vi "IMAQ Convert ROI to Oval.vi"(7 "error in (no error)":errorcluster, 10 "ROI Descriptor":T1 {"Contours"."Type" items=["No Selection", "Point", "Line", "Rectangle", "Oval", "Polygon", "Freehand Region", "Annulus", "Unused2", "Unused3", "Broken Line", "Freehand Line", "Rotated Rectangle"]}) -> (0 "error out":errorcluster, 3 "Annulus":T2 {"End Angle" min=-90.0 max=90.0 step=1.0 format="%.2f"; "Start Angle" min=-90.0 max=90.0 step=1.0 format="%.2f"; "Center X" scale=0.0..1024.0})   [LabVIEW 2013]
doc: "Converts an ROI Descriptor to an annulus."
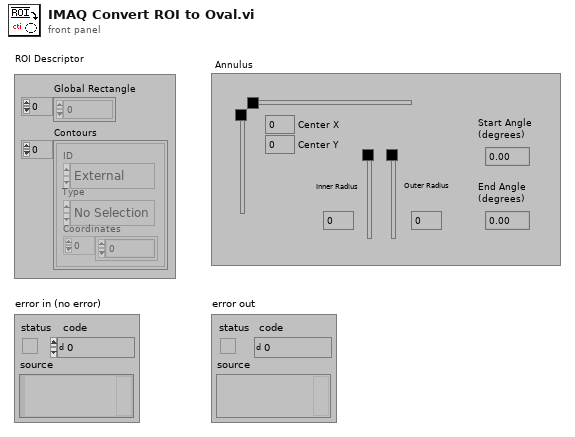
[diagram p1: front panel]
types:
  T1 = typedef "ROI Descriptor" = cluster{"Global Rectangle":i32[], "Contours":cluster{"ID":enum32{"External", "Internal"}, "Type":u32, "Coordinates":i32[]}[]}
  T2 = typedef "IMAQ Circle" = cluster{"Center X":i32, "Center Y":i32, "Inner Radius":i32, "Outer Radius":i32, "Start Angle":dbl, "End Angle":dbl}
  T3 = cluster{"ID":enum32{"External", "Internal"}, "Type":u32, "Coordinates":i32[]}[]
  T4 = cluster{"ID":enum32{"External", "Internal"}, "Type":u32, "Coordinates":i32[]}
  T5 = cluster{"Coordinates[0]":i32, "Coordinates[1]":i32, "Coordinates[2]":i32, "Coordinates[3]":i32, "Coordinates[4]":i32, "Coordinates[5]":i32}
  T6 = cluster{"Coordinates[0]":i32, "Coordinates[1]":i32, "Coordinates[2]":i32, "Coordinates[3]":i32, dbl, dbl}
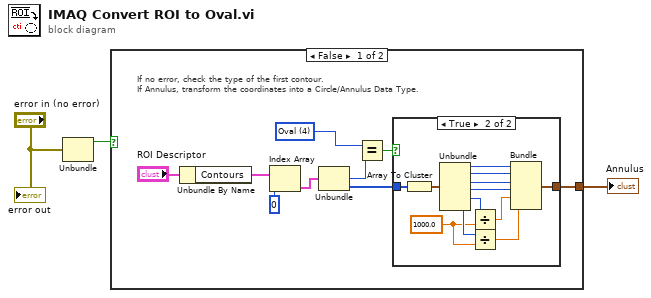
[diagram p0: block diagram]
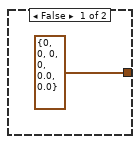
[diagram p2: hidden frame]
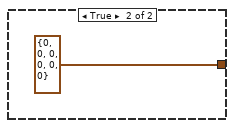
[diagram p3: hidden frame]
diagram:
  n1 = Unbundle("error in (no error)") -> ("status"=w3:bool)  [unwired: 2 out]
  n2 = case shown="False" w3 {
    tunnel: [w8 cluster{i32, i32, i32, i32, i32, i32} {0, 0, 0, 0, 0, 0} ("Coordinates")] -> w1
    frame False {
      w6 = u32 4 items=["No Selection", "Point", "Line", "Rectangle", "Oval", "Polygon", "Free", "Annulus", "Unused2", "Unused3", "Broken Line", "Free Hand Line", "Rotated Rectangle"] ("Type")
      # "If no error, check the type of the first contour.\nIf Annulus, transform the coordinates into a Circle/Annulus Data Type."
      n3 = Unbundle By Name("ROI Descriptor") -> ("Contours"=w7:T3)
      n4 = Index Array(array=w7, index=0 ("Index")) -> (element=w10:T4)
      n5 = Unbundle(w10) -> ("Type"=w5:u32, "Coordinates"=w9:i32[])  [unwired: 1 out]
      n6 = Equal?(x=w6, y=w5) -> (x = y?=w4:bool)
      n7 = case shown="True" w4 {
        tunnel: w9 -> [_ w25]
        tunnel: [cluster{i32, i32, i32, i32, dbl, dbl} {0, 0, 0, 0, 0.0, 0.0} ("Coordinates") w23] -> w8
        frame False {
        }
        frame True {
          w16 = 1000.0 ("y")
          n8 = Array To Cluster(array=w25) -> (cluster=w24:T5)
          n9 = Unbundle(w24) -> ("Coordinates[0]"=w22:i32, "Coordinates[1]"=w21:i32, "Coordinates[2]"=w20:i32, "Coordinates[3]"=w19:i32, "Coordinates[4]"=w18:i32, "Coordinates[5]"=w17:i32)
          n10 = Divide(x=w18, y=w16) -> (x/y=w15:dbl)
          n11 = Divide(x=w17, y=w16) -> (x/y=w14:dbl)
          n12 = Bundle("Coordinates[0]"=w22, "Coordinates[1]"=w21, "Coordinates[2]"=w20, "Coordinates[3]"=w19, w15, w14) -> (w23:T6)  [unwired: 1 out]
        }
      }
    }
    frame True {
    }
  }
  "Annulus" <- w1
  "error out" <- "error in (no error)"
